vi "Check - In Memory.vi"(11 "New QControl Info":refnum<data-value>) -> (0 "error out":errorcluster)   [LabVIEW 2019, in "New QControl Info.lvclass"]
doc: "<b> </b> <b> </b>\n©2016 Q Software Innovations, LLC (QSI)\nwritten by Quentin Alldredge\nproduced in LabVIEW 2015\n\nsupport@qsoftwareinnovations.com\nwww.qsoftwareinnovations.com\n\nAll rights reserved.\n\nRedistribution and use in source and binary forms, with or without modification, are permitted provided that the following conditions are met:\n\n * Redistributions of source code must retain the above copyright notice, this list of conditions and the following disclaimer.\n * Redistributions in binary form must reproduce the above copyright notice, this list of conditions and the following disclaimer in the documentation and/or other materials provided with the distribution.\n * Neither the name of Q Software Innovations, LLC. nor the names of its contributors may be used to endorse or promote products derived from this software without specific prior written permission.\n\nTHIS SOFTWARE IS PROVIDED BY THE COPYRIGHT HOLDERS AND CONTRIBUTORS \"AS IS\" AND ANY EXPRESS OR IMPLIED WARRANTIES, INCLUDING, BUT NOT LIMITED TO, THE IMPLIED WARRANTIES OF MERCHANTABILITY AND FITNESS FOR A PARTICULAR PURPOSE ARE DISCLAIMED. IN NO EVENT SHALL THE COPYRIGHT OWNER OR CONTRIBUTORS BE LIABLE FOR ANY DIRECT, INDIRECT, INCIDENTAL, SPECIAL, EXEMPLARY, OR CONSEQUENTIAL DAMAGES (INCLUDING, BUT NOT LIMITED TO, PROCUREMENT OF SUBSTITUTE GOODS OR SERVICES; LOSS OF USE, DATA, OR PROFITS; OR BUSINESS INTERRUPTION) HOWEVER CAUSED AND ON ANY THEORY OF LIABILITY, WHETHER IN CONTRACT, STRICT LIABILITY, OR TORT (INCLUDING NEGLIGENCE OR OTHERWISE) ARISING IN ANY WAY OUT OF THE USE OF THIS SOFTWARE, EVEN IF ADVISED OF THE POSSIBILITY OF SUCH DAMAGE."
uses:
  New QControl Info/New QControl Info.lvclass
  New QControl Info/New QControl Info.lvclass/New QControl Info.ctl
  New QControl Info/Read App Refnum.vi
  New QControl Info/Read QControl Class Name.vi
  <vilib>/ErrorRing/Error Ring.xnode
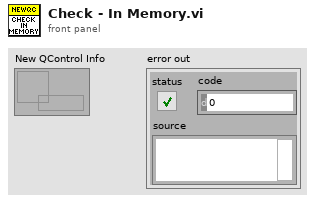
[diagram p1: front panel]
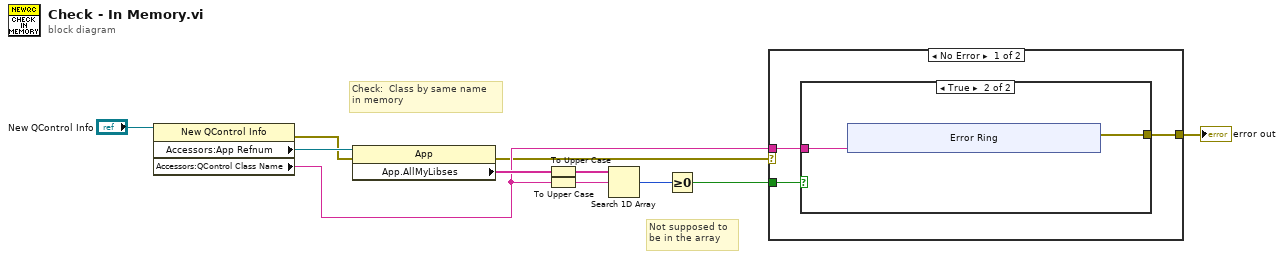
[diagram p0: block diagram]
diagram:
  # "Not supposed to\nbe in the array"
  # "Check:  Class by same name\nin memory"
  n1 = property class="New QControl Info"(reference="New QControl Info") -> (error out=w2:errorcluster, "Accessors:App Refnum"=w4:refnum<vi>, "Accessors:QControl Class Name"=w3:string)  [unwired: 1 in, 1 out]
  n2 = property class="App"(reference=w4, error in=w2) -> (error out=w1:errorcluster, "App.AllMyLibses"=w10:string[])  [unwired: 1 out]
  n3 = To Upper Case(1:w10) -> (0:w9:string[])
  n4 = To Upper Case(1:w3) -> (0:w8:string)
  n5 = Search 1D Array(1D array=w9, element=w8) -> (index of element=w11:i32)  [unwired: 1 in]
  n6 = Greater Or Equal To 0?(x=w11) -> (x >= 0?=w7:bool)
  n7 = case shown="No Error" w1 {
    selector: w1 -> [_ w22]
    tunnel: w7 -> [w14 _]
    tunnel: [w13 w22] -> w6
    tunnel: w3 -> [w12 _]
    frame No Error {
      n8 = case shown="True" w14 {
        tunnel: w12 -> [_ w16]
        tunnel: [_ w15] -> w13
        frame False {
        }
        frame True {
          n9 = xnode "Error Ring"("parameter 0"=w16) -> ("error out"=w15:errorcluster)
        }
      }
    }
    frame Error {
    }
  }
  "error out" <- w6
